vi "Decrease_Statuses_Connect_Dots_with_111-1.vi"(6 "[IN] Subtracks":T2(array[cluster]), 7 "[IN] Still connected\ntracks in group":T1, 8 "error IN":errorcluster, 9 "[IN] Decrease Statuses \nof Connected Dots":bool, 10 "[IN] Clusters for Re\nconstructed Tracks":T3) -> (0 "error OUT":errorcluster, 2 "[OUT] Clusters for Re\nconstructed Tracks":T3)   [LabVIEW 2013]
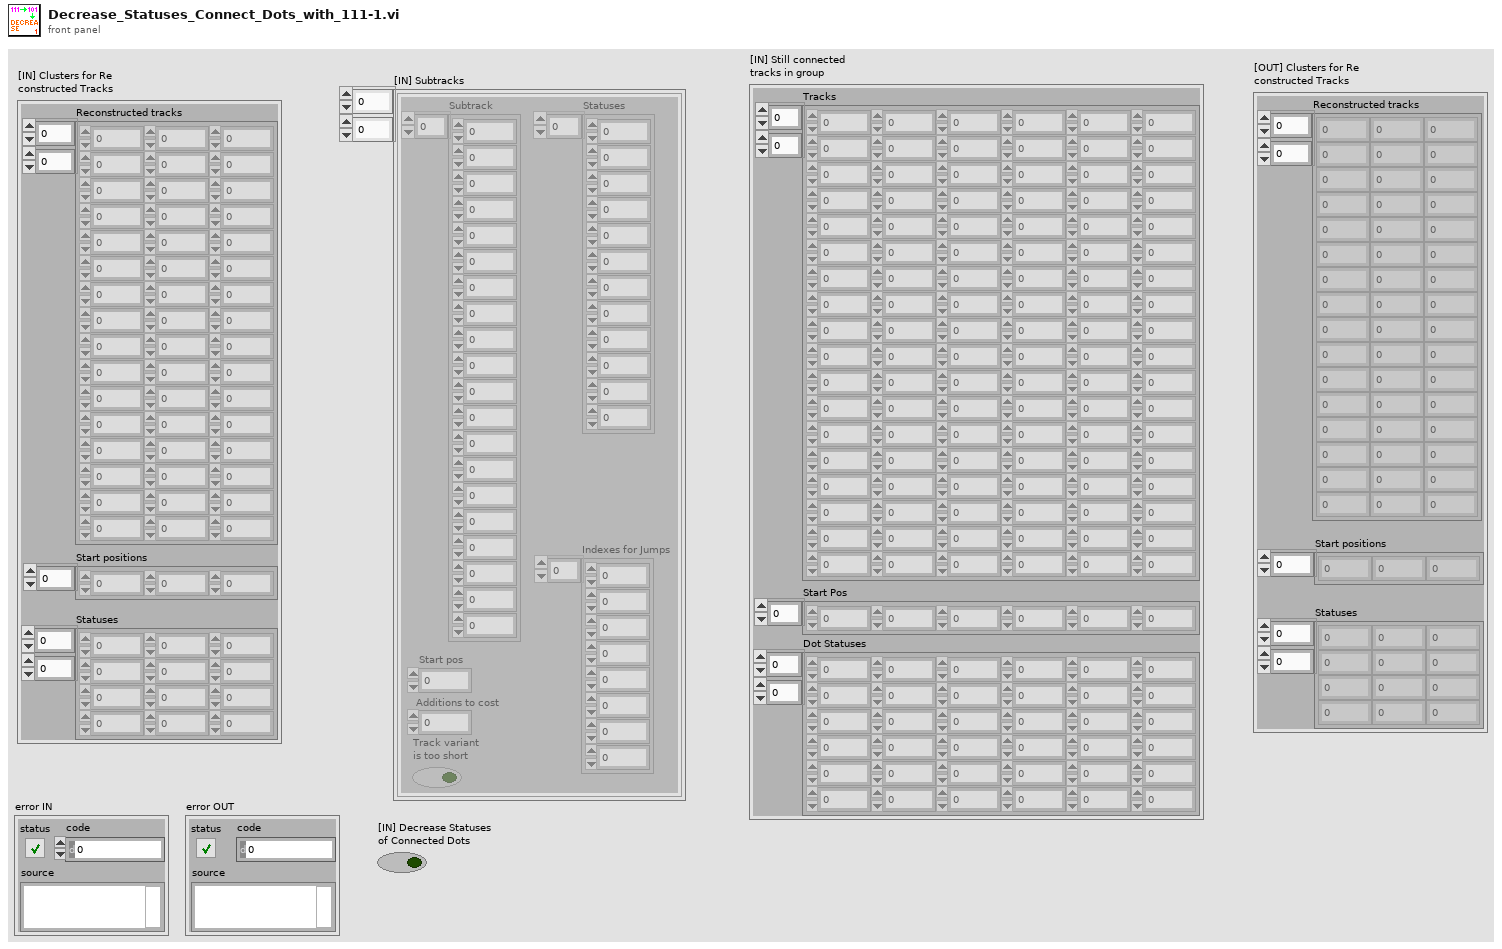
[diagram p1: front panel]
types:
  T1 = cluster{"Tracks":dbl[][], "Start Pos":i32[], "Dot Statuses":i16[][]}
  T2 = cluster{"Subtrack":dbl[], "Statuses":i16[], "Start pos":i32, "Additions to cost":i32, "Track variant \nis too short":bool, "Indexes for Jumps":i32[]}[][]
  T3 = cluster{"Reconstructed tracks":dbl[][], "Start positions":i32[], "Statuses":i16[][]}
  T4 = cluster{"Subtrack":dbl[], "Statuses":i16[], "Start pos":i32, "Additions to cost":i32, "Track variant \nis too short":bool, "Indexes for Jumps":i32[]}[]
  T5 = cluster{"Subtrack":dbl[], "Statuses":i16[], "Start pos":i32, "Additions to cost":i32, "Track variant \nis too short":bool, "Indexes for Jumps":i32[]}
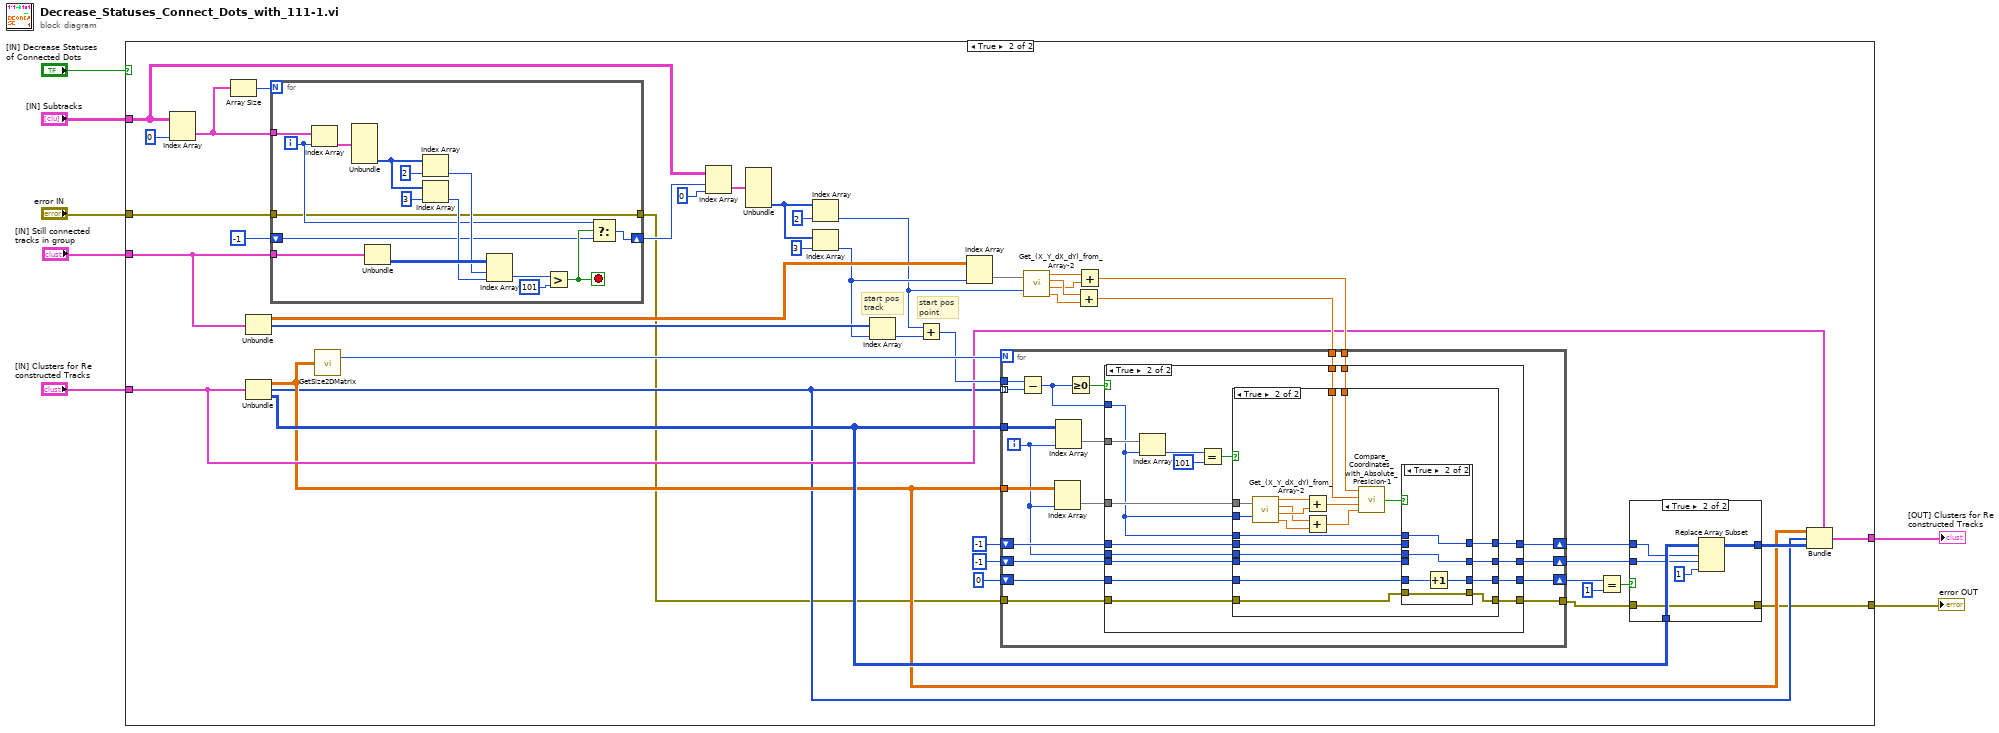
[diagram p0: block diagram]
diagram:
  n1 = case shown="True" "[IN] Decrease Statuses \nof Connected Dots" {
    tunnel: "[IN] Subtracks" -> [_ w46]
    tunnel: "[IN] Still connected\ntracks in group" -> [_ w50]
    tunnel: "[IN] Clusters for Re\nconstructed Tracks" -> [w9 w18]
    tunnel: "error IN" -> [w8 w14]
    tunnel: [w9 w12] -> w2
    tunnel: [w8 w10] -> w1
    frame False {
    }
    frame True {
      # "start pos\npoint"
      # "start pos\ntrack"
      n2 = Index Array(array=w46, index (col)=0 ("disabled index (col)")) -> (element=w51:T4)  [unwired: 1 in]
      n3 = Array Size(array=w51) -> (size(s)=w52:i32)
      n4 = Unbundle(w50) -> ("Tracks"=w37:dbl[][], "Start Pos"=w40:i32[])  [unwired: 1 out]
      n5 = Unbundle(w18) -> ("Reconstructed tracks"=w16:dbl[][], "Start positions"=w15:i32[], "Statuses"=w22:i16[][])
      n6 = for {
        N: w52 -> [_]
        tunnel: w51 -> [w151]
        tunnel: w50 -> [w146]
        shift-right: [w137] -> w45
        shift-left: -1 -> [w138]
        tunnel: w14 -> [w136]
        tunnel: [w136] -> w13
        i -> [w139]
        stop <- w141 stop-if-true
        n7 = Index Array(array=w151, index=w139) -> (element=w150:T5)
        n8 = Unbundle(w150) -> ("Indexes for Jumps"=w147:i32[])  [unwired: 5 out]
        n9 = Unbundle(w146) -> ("Dot Statuses"=w145:i16[][])  [unwired: 2 out]
        n10 = Index Array(array=w147, index=2) -> (element=w142:i32)
        n11 = Index Array(array=w147, index=3) -> (element=w140:i32)
        n12 = Index Array(array=w145, index (row)=w142, index (col)=w140) -> (element=w144:i16)
        n13 = Greater?(x=w144, y=i16 101) -> (0:w141:bool)
        n14 = Select(t=w139, s=w141, f=w138) -> (s? t:f=w137:i32)
      }
      n15 = call "GetSize2DMatrix.vi"("Array IN (2D)"=w16) -> ("# Cols"=w48:i32)  [unwired: 1 out]
      n16 = Index Array(array=w46, index (row)=w45, index (col)=0 ("disabled index (col)")) -> (element=w44:T5)
      n17 = Unbundle(w44) -> ("Indexes for Jumps"=w41:i32[])  [unwired: 5 out]
      n18 = Index Array(array=w41, index=2) -> (element=w34:i32)
      n19 = Index Array(array=w41, index=3) -> (element=w36:i32)
      n20 = Index Array(array=w40, index=w36) -> (element=w39:i32)
      n21 = Add(x=w34, y=w39) -> (x+y=w38:i32)
      n22 = Index Array(array=w37, index (col)=w36) -> (element=w35:dbl[])  [unwired: 1 in]
      n23 = call "Get_(X_Y_dX_dY)_from_Array-2.vi"("(X,Y,dX,dY)"=w35, "Index of Displacement"=w34) -> ("X"=w33:dbl, "Y"=w32:dbl, "dX"=w31:dbl, "dY"=w30:dbl)
      n24 = Add(x=w32, y=w30) -> (x+y=w28:dbl)
      n25 = Add(x=w33, y=w31) -> (x+y=w29:dbl)
      n26 = for {
        N: w48 -> [_]
        tunnel: w15 -> [w80] mode=indexing
        tunnel: w38 -> [w79]
        tunnel: w16 -> [w75]
        tunnel: w29 -> [w73]
        tunnel: w28 -> [w72]
        tunnel: w22 -> [w71]
        shift-right: [w69] -> w24
        shift-left: 0 -> [w70]
        shift-right: [w65] -> w20
        shift-left: -1 -> [w67]
        shift-right: [w64] -> w21
        shift-left: -1 -> [w68]
        tunnel: w13 -> [w63]
        tunnel: [w62] -> w11
        i -> [w66]
        n27 = Subtract(x=w79, y=w80) -> (x-y=w77:i32)
        n28 = Index Array(array=w75, index (col)=w66) -> (element=w74:dbl[])  [unwired: 1 in]
        n29 = Index Array(array=w71, index (col)=w66) -> (element=w76:i16[])  [unwired: 1 in]
        n30 = Greater Or Equal To 0?(x=w77) -> (x >= 0?=w78:bool)
        n31 = case shown="True" w78 {
          tunnel: w77 -> [_ w90]
          tunnel: w76 -> [_ w101]
          tunnel: w74 -> [_ w97]
          tunnel: w73 -> [_ w96]
          tunnel: w72 -> [_ w95]
          tunnel: w70 -> [w84 w94]
          tunnel: [w84 w93] -> w69
          tunnel: w68 -> [w82 w92]
          tunnel: w67 -> [w83 w91]
          tunnel: w66 -> [_ w89]
          tunnel: [w83 w88] -> w65
          tunnel: [w82 w87] -> w64
          tunnel: w63 -> [w81 w86]
          tunnel: [w81 w85] -> w62
          frame False {
          }
          frame True {
            n32 = Index Array(array=w101, index=w90) -> (element=w100:i16)
            n33 = Equal?(x=w100, y=i16 101) -> (x = y?=w98:bool)
            n34 = case shown="True" w98 {
              tunnel: w97 -> [_ w126]
              tunnel: w90 -> [_ w125]
              tunnel: w96 -> [_ w118]
              tunnel: w95 -> [_ w117]
              tunnel: w94 -> [w104 w115]
              tunnel: [w104 w114] -> w93
              tunnel: w92 -> [w103 w113]
              tunnel: w91 -> [w105 w112]
              tunnel: w90 -> [_ w111]
              tunnel: w89 -> [_ w110]
              tunnel: [w105 w109] -> w88
              tunnel: [w103 w108] -> w87
              tunnel: w86 -> [w102 w107]
              tunnel: [w102 w106] -> w85
              frame False {
              }
              frame True {
                n35 = call "Get_(X_Y_dX_dY)_from_Array-2.vi"("(X,Y,dX,dY)"=w126, "Index of Displacement"=w125) -> ("X"=w124:dbl, "Y"=w122:dbl, "dX"=w123:dbl, "dY"=w121:dbl)
                n36 = Add(x=w124, y=w123) -> (x+y=w120:dbl)
                n37 = Add(x=w122, y=w121) -> (x+y=w119:dbl)
                n38 = call "Compare_Coordinates_with_Absolute_Presicion-1.vi"("X 1"=w118, "Y 1"=w117, "X 2"=w120, "Y 2"=w119) -> ("[OUT] Same coordinates?"=w116:bool)  [unwired: 1 in]
                n39 = case shown="True" w116 {
                  tunnel: w115 -> [w130 w135]
                  tunnel: [w130 w134] -> w114
                  tunnel: w113 -> [w128 _]
                  tunnel: w112 -> [w129 _]
                  tunnel: [w129 w133] -> w109
                  tunnel: [w128 w132] -> w108
                  tunnel: w111 -> [_ w133]
                  tunnel: w110 -> [_ w132]
                  tunnel: w107 -> [w127 w131]
                  tunnel: [w127 w131] -> w106
                  frame False {
                  }
                  frame True {
                    n40 = Increment(x=w135) -> (x+1=w134:i32)
                  }
                }
              }
            }
          }
        }
      }
      n41 = Equal?(x=w24, y=1) -> (x = y?=w19:bool)
      n42 = case shown="True" w19 {
        tunnel: w22 -> [w55 w61]
        tunnel: w21 -> [_ w60]
        tunnel: w20 -> [_ w59]
        tunnel: [w55 w57] -> w17
        tunnel: w11 -> [w54 w56]
        tunnel: [w54 w56] -> w10
        frame False {
        }
        frame True {
          n43 = Replace Array Subset(array=w61, new element=i16 1 ("new element/subarray"), index (row)=w59, index (col)=w60) -> (w57:i16[][])
        }
      }
      n44 = Bundle(cluster=w18, "Reconstructed tracks"=w16, "Start positions"=w15, "Statuses"=w17) -> (w12:T3)
    }
  }
  "[OUT] Clusters for Re\nconstructed Tracks" <- w2
  "error OUT" <- w1
